vi "Eliminated.vi"(6 "Column":i32, 8 "Row":i32, 9 "Killer":i32, 10 "Team":i32, 11 "Team 3 in":refnum<class "Team 3.lvclass">) -> (3 "Team 3 out":refnum<class "Team 3.lvclass">)   [LabVIEW 2020, in "Team 3.lvclass"]
uses:
  Team 3.lvclass
  Team 3.lvclass/Team 3.ctl
  Square/Square.lvclass
  DS Square Library/DS Square.lvlib
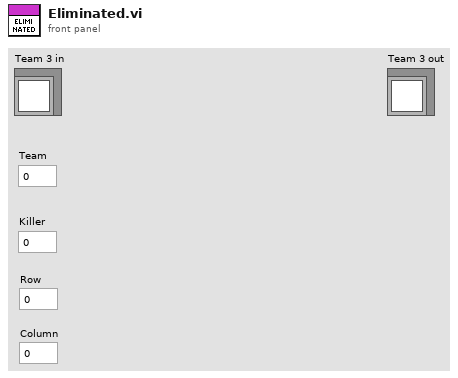
[diagram p1: front panel]
types:
  T1 = typedef "Common.lvlib/Position.ctl" = cluster{"Column":i32, "Row":i32}
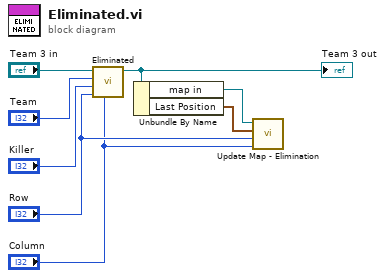
[diagram p0: block diagram]
diagram:
  n1 = call-parent "Eliminated.vi"("Column"="Column", "Row"="Row", "Killer Index"="Killer", "Team Index"="Team", "Square in"="Team 3 in") -> ("Square out"=w5:refnum<class "Team 3.lvclass">)  [unwired: 6 in]
  "Team 3 out" <- w5
  n2 = Unbundle By Name(w5) -> ("map in"=w4:refnum<data-value>, "Last Position"=w1:T1)
  n3 = call "Update Map - Elimination.vi"("Column"="Column", "Row"="Row", "Last Position"=w1, "map in"=w4) -> ()  [unwired: 7 in, 1 out]
